vi "FlatToRichrfcontrol_SCPICommandRequest.vi"(5 "OutputClusterType":T1, 11 "InputCluster":T2) -> (3 "OutputCluster":T1)   [LabVIEW 2024, in "FlexSDR_gRPC_client.lvlib"]
uses:
  rfcontrol_SCPICommandRequest_Flat.ctl
  rfcontrol_SCPICommandRequest.ctl
  FlexSDR_gRPC_client.lvlib
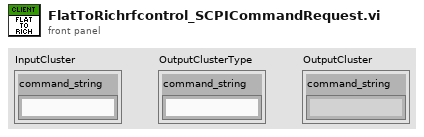
[diagram p1: front panel]
types:
  T1 = typedef "FlexSDR_gRPC_client.lvlib/rfcontrol_SCPICommandRequest.ctl" = cluster{"command_string":string}
  T2 = typedef "FlexSDR_gRPC_client.lvlib/rfcontrol_SCPICommandRequest_Flat.ctl" = cluster{"command_string":string}
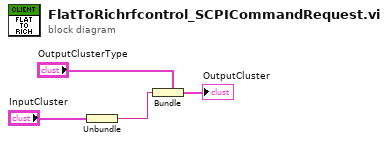
[diagram p0: block diagram]
diagram:
  n1 = Unbundle "Unbundle"("InputCluster") -> ("command_string"=w1:string)
  n2 = Bundle "Bundle"(cluster="OutputClusterType", "command_string"=w1) -> (→"OutputCluster":T1)
